vi "Read Operator Joystick.vi"   [LabVIEW 2020]
uses:
  <vilib>/Rock Robotics/WPI/Utilities/WPI_GetSetVariantRefNum.vi
  Framework/Robot Global Data.vi
  <vilib>/Rock Robotics/Network Tables/NT Write Numeric Array.vi
  <vilib>/Rock Robotics/Network Tables/NT Write Boolean Array.vi
types:
  T1 = enum16{"0", "1", "2", "3", "4", "5", "6", "7", "8", "9", "10", "11"}
  T2 = typedef "WPI_JoystickDevRef.ctl" = cluster{"Device":T3}
  T3 = typedef "WPI_JoystickDeviceEnum.ctl" = enum16{"USB 0", "USB 1", "USB 2", "USB 3", "USB 4", "USB 5"}
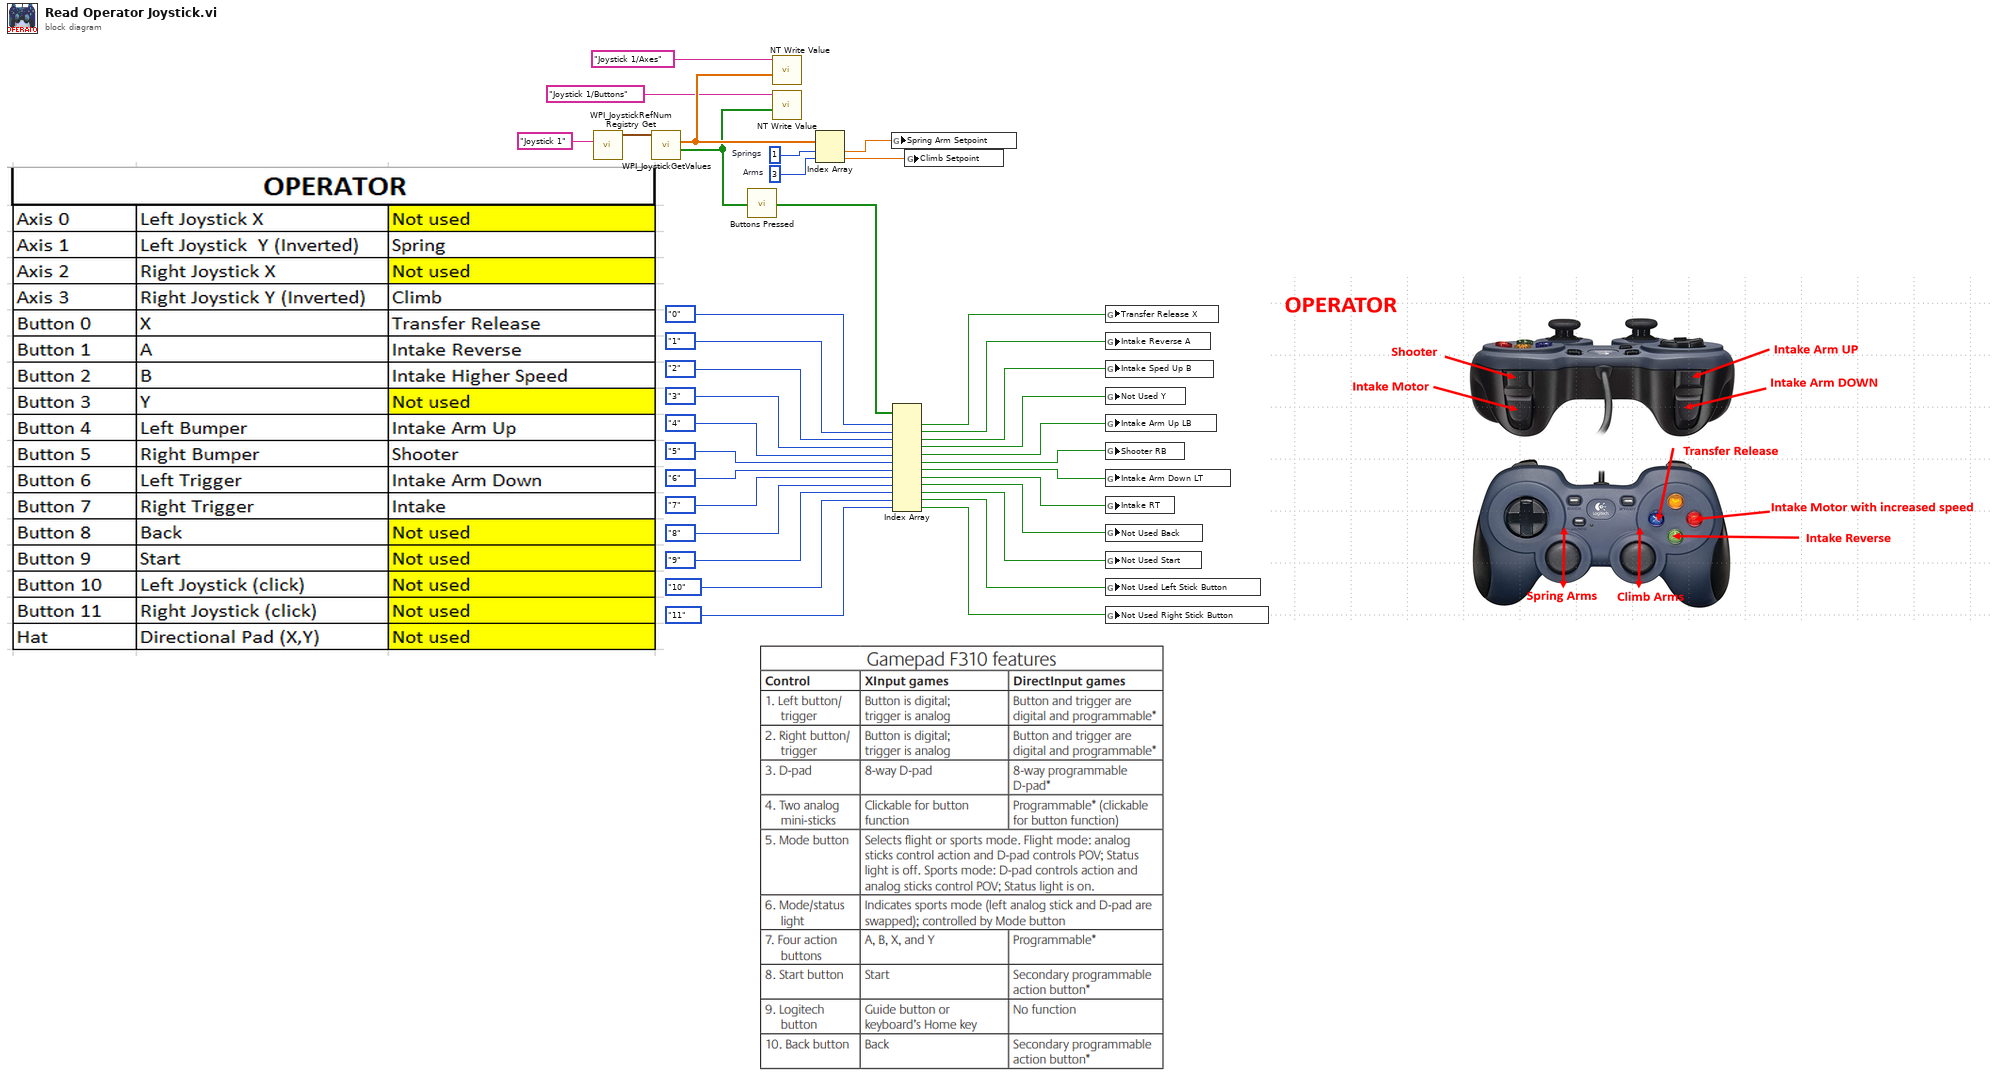
[diagram p0: block diagram]
diagram:
  w32 = 3  # Arms
  w33 = 1  # Springs
  n1 = call <vilib>:"WPI_JoystickRefNum Registry Get.vi"("refnum name"="Joystick 1") -> ("JoystickDevRef"=w35:T2)  [unwired: 9 in, 1 out]
  n2 = call <vilib>:"WPI_JoystickGetValues.vi"("JoystickDevRef"=w35) -> ("Buttons"=w30:bool[], "Axes"=w31:dbl[])  [unwired: 6 in, 3 out]
  n3 = call "Buttons Pressed.vi"("Button Values"=w30) -> ("Button Presses"=w29:bool[])
  n4 = call-poly <vilib>:"NT Write Value.vi"("Numeric Array"=w31, "Name"="Joystick 1/Axes") -> ()  [unwired: 9 in, 1 out]
  n5 = call-poly <vilib>:"NT Write Value.vi"("Boolean Array"=w30, "Name"="Joystick 1/Buttons") -> ()  [unwired: 9 in, 1 out]
  n6 = Index Array(array=w31, index #1=w33, index #2=w32) -> (element #1=w28:dbl, element #2=w27:dbl)
  n7 = global write "Robot Global Data.vi" "Spring Arm Setpoint"(w28) -> ()
  n8 = Index Array(array=w29, index #1=T1."0", index #2=T1."1", index #3=T1."2", index #4=T1."3", index #5=T1."4", index #6=T1."5", index #7=T1."6", index #8=T1."7", index #9=T1."8", index #10=T1."9", index #11=T1."10", index #12=T1."11") -> (element #1=w22:bool, element #2=w21:bool, element #3=w20:bool, element #4=w19:bool, element #5=w17:bool, element #6=w14:bool, element #7=w12:bool, element #8=w8:bool, element #9=w7:bool, element #10=w3:bool, element #11=w2:bool, element #12=w1:bool)
  n9 = global write "Robot Global Data.vi" "Climb Setpoint"(w27) -> ()
  n10 = global write "Robot Global Data.vi" "Transfer Release X"(w22) -> ()
  n11 = global write "Robot Global Data.vi" "Intake Reverse A"(w21) -> ()
  n12 = global write "Robot Global Data.vi" "Intake Sped Up B"(w20) -> ()
  n13 = global write "Robot Global Data.vi" "Not Used Y"(w19) -> ()
  n14 = global write "Robot Global Data.vi" "Intake Arm Up LB"(w17) -> ()
  n15 = global write "Robot Global Data.vi" "Shooter RB"(w14) -> ()
  n16 = global write "Robot Global Data.vi" "Intake Arm Down LT"(w12) -> ()
  n17 = global write "Robot Global Data.vi" "Intake RT"(w8) -> ()
  n18 = global write "Robot Global Data.vi" "Not Used Back"(w7) -> ()
  n19 = global write "Robot Global Data.vi" "Not Used Start"(w3) -> ()
  n20 = global write "Robot Global Data.vi" "Not Used Left Stick Button"(w2) -> ()
  n21 = global write "Robot Global Data.vi" "Not Used Right Stick Button"(w1) -> ()
